vi "HEWH Extract Str Data.vi"(7 "Full Data (String)":string[][](array[string]), 8 "error in (no error)":errorcluster, 11 "UEF Calculated Values Input in":T1 {"Data Indexes"."15 sec after Draw Index" format="%#.2f"; "Data Indexes"."15 sec after Draw Timestamp" format="%#.2f"; "Data Indexes"."Test Start Timestamp" format="%.2f"; "Data Indexes"."Test End Timestamp" format="%.2f"; "Data Indexes"."T0 Timestamp" format="%.2f"; "Data Indexes"."Tsf Timestamp" format="%.2f"; "Data Indexes"."Tsu0 Timestamp" format="%.2f"; "Data Indexes"."Tmax1 Timestamp" format="%.2f"; "Data Indexes"."Draw Index Timestamp" format="%#.2f"; "Data Indexes"."Non-Draw Timestamp" format="%#.2f"; "Data Indexes"."Heating Timestamp" format="%#.2f"; "Data Indexes"."Start Energy (BTU-Gas)" format="%.6f"; "Data Indexes"."Start Watt Hours" format="%.6f"; "Static Data"."V - Volume of Wh (True)" format="%.5f"; "Static Data"."T-Ambinet Nominal (°F)" format="%.5f"; "Static Data"."T-Inlet Setpoint (°F)" format="%.5f"; "Static Data"."T-Wh Setpoint (°F)" format="%.5f"; "Sampled Data"."Qe (Wh)" format="%.5f"; "Sampled Data"."Tau stby2 (hr)" format="%.5f"; "Sampled Data"."Tastby2 (°F)" format="%.5f"; "Sampled Data"."Qf (BTU)" format="%.5f"; "Sampled Data"."Qe (BTU)" format="%.5f"; "Sampled Data"."Tmax1 (°F)" format="%.5f"; "Sampled Data"."T0 (°F)" format="%.5f"; "Sampled Data"."Qr (BTU)" format="%.5f"; "Sampled Data"."T 24(°F)" format="%.5f"; "Sampled Data"."T astby(°F)" format="%.5f"; "Sampled Data"."T tstby(°F)" format="%.5f"; "Sampled Data"."T su0(°F)" format="%.5f"; "Sampled Data"."T suf(°F)" format="%.5f"; "Sampled Data"."Tau stby_1 (hr)" format="%.5f"; "Sampled Data"."Qsuf (BTU)" format="%.5f"; "Sampled Data"."Qsu0 (BTU)" format="%.5f"; "Calculated Values"."Draw Bonus Volume (gal)" format="%.6f"; "Calculated Values"."Adjustment Factor" format="%.6f"; "Calculated Values"."T*avg_del(n-1)" format="%.6f"; "Calculated Values"."T*min(n-1)" format="%.6f"; "Calculated Values"."T*avg_del(n)" format="%.6f"; "Calculated Values"."Vn" format="%.6f"; "Calculated Values"."Qdm (BTU)" format="%.6f"; "Calculated Values"."QHWD (BTU)" format="%.6f"; "Calculated Values"."QHW (BTU)" format="%.6f"; "Calculated Values"."UEF" format="%.6f"; "Calculated Values"."QHW67 (BTU)" format="%.6f"; "Calculated Values"."Qda (BTU)" format="%.6f"; "Calculated Values"."Qd (BTU)" format="%.6f"; "Calculated Values"."Q (BTU)" format="%.6f"; "Calculated Values"."UA (BTU/(hr*F))" format="%.6f"; "Calculated Values"."Qhr (BTU/hr)" format="%.6f"; "Calculated Values"."Qstby (BTU)" format="%.6f"; "Calculated Values"."nu_r" format="%.6f"; "Calculated Values"."CpUEF (BTU/(lb*F))" format="%.6f"; "Calculated Values"."rho_nu (lb/gal)" format="%.6f"; "Calculated Values"."V1- Vol (Gal)" format="%.6f"; "Calculated Values"."M cluster mass removed (lb)" format="%.6f"; "Calculated Values"."Cp theoretical (BTU/(lbm °F))" format="%.6f"; "Calculated Values"."Tin1 - Mean Inlet 1st Cluster (°F)" format="%.6f"; "Calculated Values"."Tdel1-Mean Outlet 1st Cluster(°F)" format="%.6f"; "Calculated Values"."Cp 24 (BTU/(lb*F))" format="%.6f"; "Calculated Values"."Cp standby (BTU/(lb*F))" format="%.6f"; "Calculated Values"."Cp2 (BTU/(lb*F))" format="%.6f"; "Calculated Values"."Cp1 (BTU/(lb*F))" format="%.6f"; "Calculated Values"."rho 24 (lb/gal)" format="%.6f"; "Calculated Values"."rho standby (lb/gal)" format="%.6f"; "Calculated Values"."rho 2 (lb/gal)" format="%.6f"; "Calculated Values"."Density of cold water All (lbm/gal)" format="%#.3g"; "Calculated Values"."CpHW (BTU/(lbm °F))" format="%#.3g"; "Calculated Values"."Density of hot water All (lbm/gal)" format="%#.3g"; "Calculated Values"."Mass of water All (lbm)" format="%#.3f"}) -> (0 "error out":errorcluster, 1 "Full Data (String) Out":string[][](array[string]), 3 "UEF Calculated Values Input out":T1 {"Data Indexes"."15 sec after Draw Index" format="%#.2f"; "Data Indexes"."15 sec after Draw Timestamp" format="%#.2f"; "Data Indexes"."Test Start Timestamp" format="%.2f"; "Data Indexes"."Test End Timestamp" format="%.2f"; "Data Indexes"."T0 Timestamp" format="%.2f"; "Data Indexes"."Tsf Timestamp" format="%.2f"; "Data Indexes"."Tsu0 Timestamp" format="%.2f"; "Data Indexes"."Tmax1 Timestamp" format="%.2f"; "Data Indexes"."Draw Index Timestamp" format="%#.2f"; "Data Indexes"."Non-Draw Timestamp" format="%#.2f"; "Data Indexes"."Heating Timestamp" format="%#.2f"; "Data Indexes"."Start Energy (BTU-Gas)" format="%.6f"; "Data Indexes"."Start Watt Hours" format="%.6f"; "Static Data"."V - Volume of Wh (True)" format="%.5f"; "Static Data"."T-Ambinet Nominal (°F)" format="%.5f"; "Static Data"."T-Inlet Setpoint (°F)" format="%.5f"; "Static Data"."T-Wh Setpoint (°F)" format="%.5f"; "Sampled Data"."Qe (Wh)" format="%.5f"; "Sampled Data"."Tau stby2 (hr)" format="%.5f"; "Sampled Data"."Tastby2 (°F)" format="%.5f"; "Sampled Data"."Qf (BTU)" format="%.5f"; "Sampled Data"."Qe (BTU)" format="%.5f"; "Sampled Data"."Tmax1 (°F)" format="%.5f"; "Sampled Data"."T0 (°F)" format="%.5f"; "Sampled Data"."Qr (BTU)" format="%.5f"; "Sampled Data"."T 24(°F)" format="%.5f"; "Sampled Data"."T astby(°F)" format="%.5f"; "Sampled Data"."T tstby(°F)" format="%.5f"; "Sampled Data"."T su0(°F)" format="%.5f"; "Sampled Data"."T suf(°F)" format="%.5f"; "Sampled Data"."Tau stby_1 (hr)" format="%.5f"; "Sampled Data"."Qsuf (BTU)" format="%.5f"; "Sampled Data"."Qsu0 (BTU)" format="%.5f"; "Calculated Values"."Draw Bonus Volume (gal)" format="%.6f"; "Calculated Values"."Adjustment Factor" format="%.6f"; "Calculated Values"."T*avg_del(n-1)" format="%.6f"; "Calculated Values"."T*min(n-1)" format="%.6f"; "Calculated Values"."T*avg_del(n)" format="%.6f"; "Calculated Values"."Vn" format="%.6f"; "Calculated Values"."Qdm (BTU)" format="%.6f"; "Calculated Values"."QHWD (BTU)" format="%.6f"; "Calculated Values"."QHW (BTU)" format="%.6f"; "Calculated Values"."UEF" format="%.6f"; "Calculated Values"."QHW67 (BTU)" format="%.6f"; "Calculated Values"."Qda (BTU)" format="%.6f"; "Calculated Values"."Qd (BTU)" format="%.6f"; "Calculated Values"."Q (BTU)" format="%.6f"; "Calculated Values"."UA (BTU/(hr*F))" format="%.6f"; "Calculated Values"."Qhr (BTU/hr)" format="%.6f"; "Calculated Values"."Qstby (BTU)" format="%.6f"; "Calculated Values"."nu_r" format="%.6f"; "Calculated Values"."CpUEF (BTU/(lb*F))" format="%.6f"; "Calculated Values"."rho_nu (lb/gal)" format="%.6f"; "Calculated Values"."V1- Vol (Gal)" format="%.6f"; "Calculated Values"."M cluster mass removed (lb)" format="%.6f"; "Calculated Values"."Cp theoretical (BTU/(lbm °F))" format="%.6f"; "Calculated Values"."Tin1 - Mean Inlet 1st Cluster (°F)" format="%.6f"; "Calculated Values"."Tdel1-Mean Outlet 1st Cluster(°F)" format="%.6f"; "Calculated Values"."Cp 24 (BTU/(lb*F))" format="%.6f"; "Calculated Values"."Cp standby (BTU/(lb*F))" format="%.6f"; "Calculated Values"."Cp2 (BTU/(lb*F))" format="%.6f"; "Calculated Values"."Cp1 (BTU/(lb*F))" format="%.6f"; "Calculated Values"."rho 24 (lb/gal)" format="%.6f"; "Calculated Values"."rho standby (lb/gal)" format="%.6f"; "Calculated Values"."rho 2 (lb/gal)" format="%.6f"; "Calculated Values"."Density of cold water All (lbm/gal)" format="%#.3g"; "Calculated Values"."CpHW (BTU/(lbm °F))" format="%#.3g"; "Calculated Values"."Density of hot water All (lbm/gal)" format="%#.3g"; "Calculated Values"."Mass of water All (lbm)" format="%#.3f"})   [LabVIEW 2023]
uses:
  Type Definitions/UEF Constants.ctl
  Type Definitions/HEWH Draw Stats.ctl
  Type Definitions/HEWH FHR Draw Type.ctl
  Type Definitions/FHR Bins.ctl
  Type Definitions/HEWH Meter Type.ctl
panel:
  # "FHR"
  # "FHR"
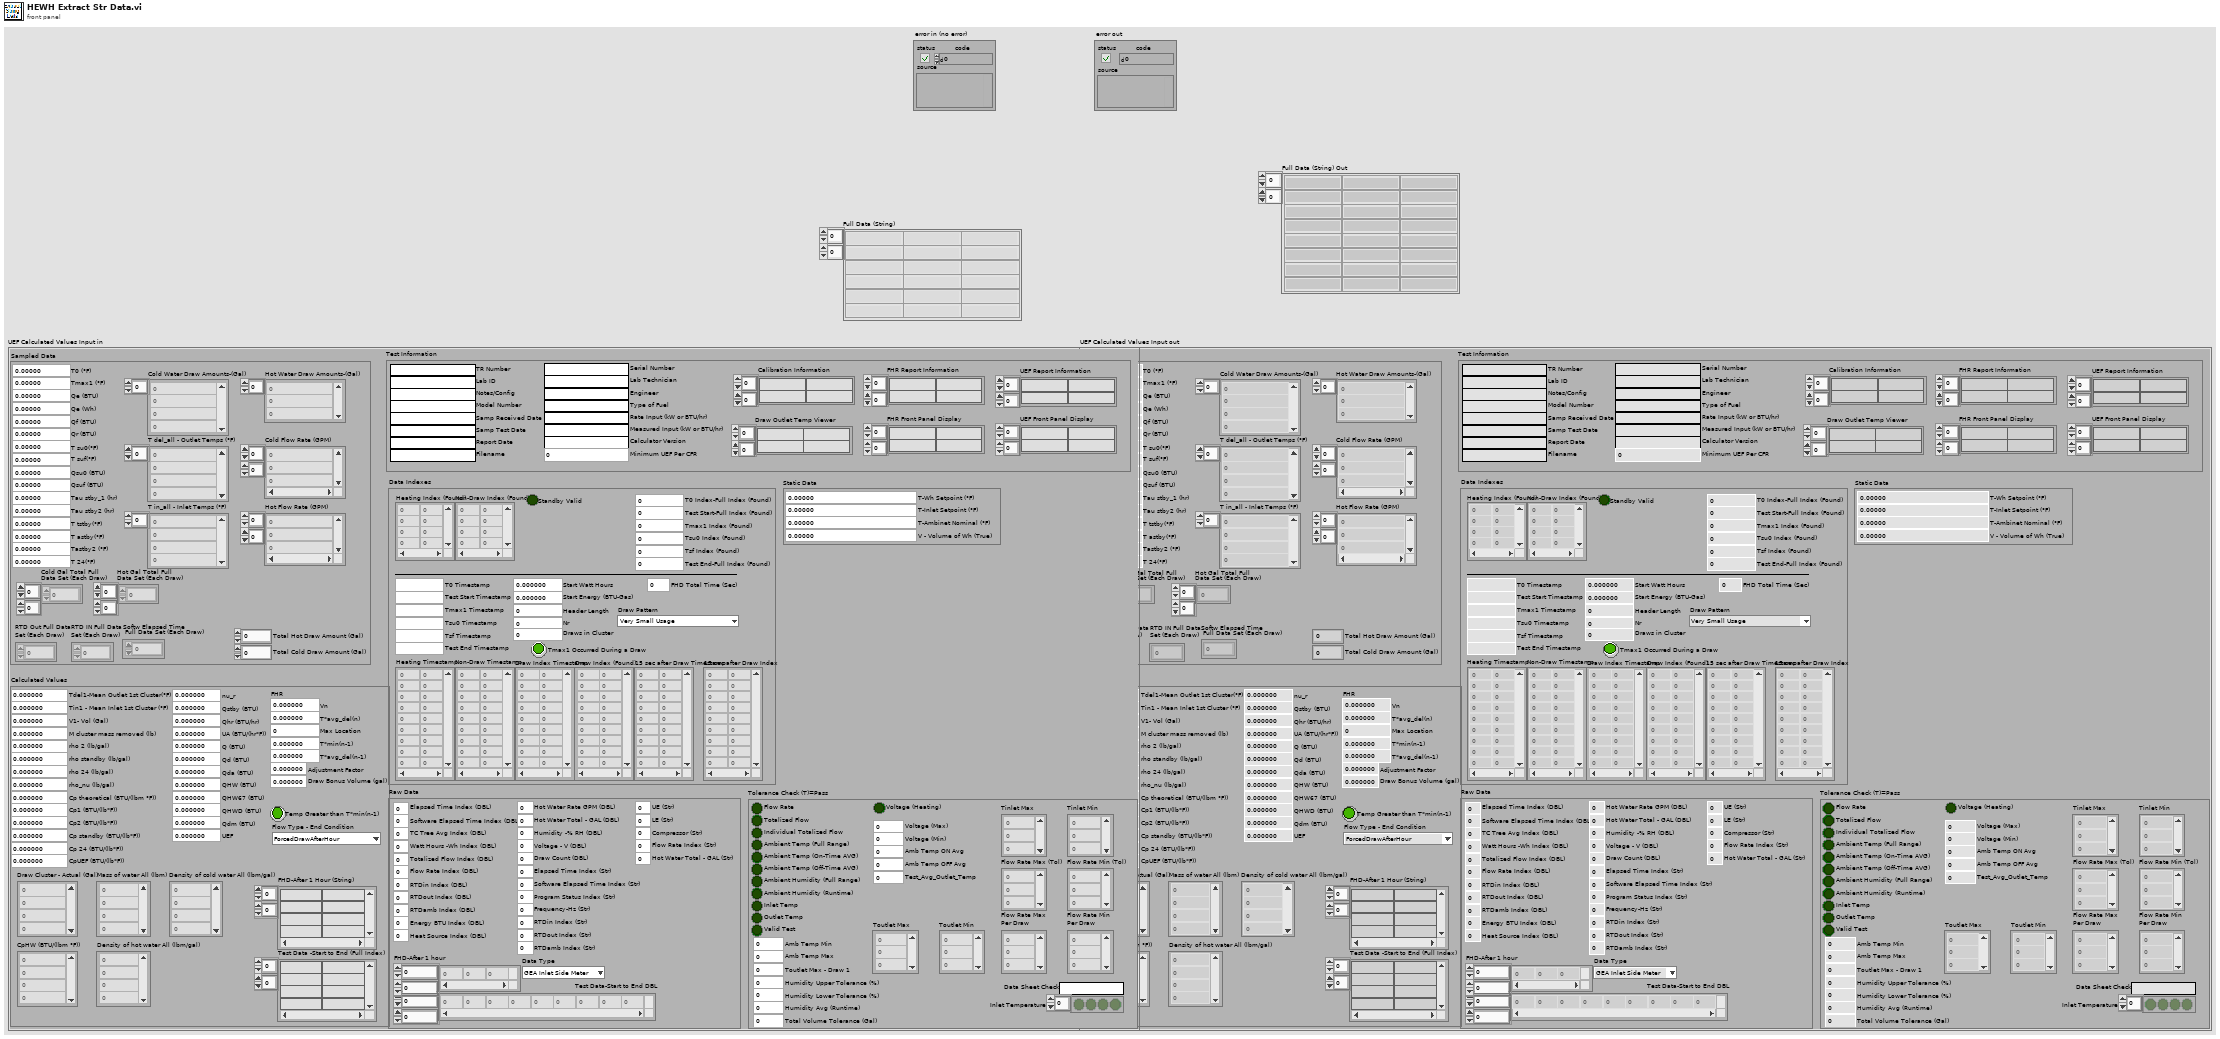
[diagram p1: front panel]
types:
  T1 = typedef "UEF Constants.ctl" = cluster{"Calculated Values":T2, "Sampled Data":cluster{"Cold Water Draw Amounts-(Gal)":dbl[], "T del_all - Outlet Temps (°F)":dbl[], "T in_all - Inlet Temps (°F)":dbl[], "Qsu0 (BTU)":dbl, "Qsuf (BTU)":dbl, "Tau stby_1 (hr)":dbl, "T suf(°F)":dbl, "T su0(°F)":dbl, "T tstby(°F)":dbl, "T astby(°F)":dbl, "T 24(°F)":dbl, "Qr (BTU)":dbl, "T0 (°F)":dbl, "Tmax1 (°F)":dbl, "Qe (BTU)":dbl, "Qf (BTU)":dbl, "Tastby2 (°F)":dbl, "RTD Out Full Data\nSet (Each Draw)":dbl[][], "RTD IN Full Data\nSet (Each Draw)":dbl[][], "Tau stby2 (hr)":dbl, "Hot Water Draw Amounts-(Gal)":dbl[], "Cold Flow Rate (GPM)":dbl[][], "Hot Flow Rate (GPM)":dbl[][], "Softw Elapsed Time\n Full Data Set (Each Draw)":dbl[][], "Cold Gal Total Full\nData Set (Each Draw)":dbl[][], "Total Hot Draw Amount (Gal) ":dbl, "Total Cold Draw Amount (Gal)":dbl, "Qe (Wh)":dbl, "Hot Gal Total Full\nData Set (Each Draw)":dbl[][]}, "Static Data":cluster{"T-Wh Setpoint (°F)":dbl, "T-Inlet Setpoint (°F)":dbl, "T-Ambinet Nominal (°F)":dbl, "V - Volume of Wh (True)":dbl}, "Data Indexes":cluster{"Test Start-Full Index (Found)":i32, "Header Length":i32, "Draw Index (Found)":i32[][], "Nr":i32, "Start Watt Hours":dbl, "Tsu0 Index (Found)":i32, "Tsf Index (Found)":i32, "Start Energy (BTU-Gas)":dbl, "Draws in Cluster":i32, "T0 Index-Full Index (Found)":i32, "Non-Draw Index (Found)":i32[][], "Tmax1 Index (Found)":i32, "Test End-Full Index (Found)":i32, "Heating Index (Found)":i32[][], "Heating Timestamp":dbl[][], "Non-Draw Timestamp":dbl[][], "Draw Index Timestamp":dbl[][], "Tmax1 Timestamp":dbl, "Tsu0 Timestamp":dbl, "Tsf Timestamp":dbl, "T0 Timestamp":dbl, "Test End Timestamp":dbl, "Test Start Timestamp":dbl, "15 sec after Draw Timestamp":dbl[][], "15 sec after Draw Index":dbl[][], "Tmax1 Occurred During a Draw":bool, "FHD Total Time (Sec)":dbl, "Draw Pattern":T4, "Standby Valid":bool}, "Raw Data":cluster{"Elapsed Time Index (DBL)":i32, "Software Elapsed Time Index (DBL)":i32, "TC Tree Avg Index (DBL)":i32, "Watt Hours -Wh Index (DBL)":i32, "Energy BTU Index (DBL)":i32, "Totalized Flow Index (DBL)":i32, "Flow Rate Index (DBL)":i32, "Program Status Index (Str)":i32, "RTDin Index (DBL)":i32, "RTDout Index (DBL)":i32, "RTDamb Index (DBL)":i32, "Test Data-Start to End DBL":dbl[][], "Data Type":T5, "Heat Source Index (DBL)":i32, "Hot Water Rate GPM (DBL)":i32, "Hot Water Total - GAL (DBL)":i32, "FHD-After 1 hour":dbl[][], "Humidity -% RH (DBL)":i32, "Voltage - V (DBL)":i32, "Draw Count (DBL)":i32, "Elapsed Time Index (Str)":i32, "Software Elapsed Time Index (Str)":i32, "Frequency-Hz (Str)":i32, "RTDin Index (Str)":i32, "RTDout Index (Str)":i32, "RTDamb Index (Str)":i32, "UE (Str)":i32, "LE (Str)":i32, "Compressor (Str)":i32, "Flow Rate Index (Str)":i32, "Hot Water Total - GAL (Str)":i32}, "Tolerance Check (T)=Pass":cluster{"Flow Rate":bool, "Totalized Flow":bool, "Ambient Temp (Full Range)":bool, "Ambient Humidity (Full Range)":bool, "Inlet Temp":bool, "Outlet Temp":bool, "Valid Test":bool, "Individual Totalized Flow":bool, "Data Sheet Check":string, "Inlet Temperature":bool[], "Tinlet Max":dbl[], "Tinlet Min":dbl[], "Flow Rate Max (Tol)":dbl[], "Flow Rate Min (Tol)":dbl[], "Amb Temp Max":dbl, "Amb Temp Min":dbl, "Toutlet Max - Draw 1":dbl, "Humidity Upper Tolerance (%)":dbl, "Total Volume Tolerance (Gal)":dbl, "Humidity Lower Tolerance (%)":dbl, "Flow Rate Max\nPer Draw":dbl[], "Flow Rate Min\nPer Draw":dbl[], "Ambient Humidity (Runtime)":bool, "Humidity Avg (Runtime)":dbl, "Ambient Temp (On-Time AVG)":bool, "Ambient Temp (Off-Time AVG)":bool, "Amb Temp OFF Avg":dbl, "Amb Temp ON Avg":dbl, "Voltage (Heating)":bool, "Voltage (Min)":dbl, "Voltage (Max)":dbl, "Toutlet Max":dbl[], "Toutlet Min":dbl[], "Test_Avg_Outlet_Temp":dbl}, "Test Information":cluster{"TR Number":string, "Lab ID":string, "Notes/Config":string, "Model Number":string, "Serial Number":string, "Lab Technician":string, "Engineer":string, "Type of Fuel":string, "Samp Received Date":string, "Samp Test Date":string, "Report Date":string, "Rate Input (kW or BTU/hr)":string, "Measured Input (kW or BTU/hr)":string, "Filename":string, "Calibration Information":string[][], "Calculator Version":string, "Minimum UEF Per CFR":dbl, "UEF Report Information":string[][], "FHR Report Information":string[][], "FHR Front Panel Display":string[][], "UEF Front Panel Display":string[][], "Draw Outlet Temp Viewer":string[][]}}
  T2 = typedef "HEWH Draw Stats.ctl" = cluster{"Draw Cluster - Actual (Gal)":dbl[], "Mass of water All (lbm)":dbl[], "Density of hot water All (lbm/gal)":dbl[], "CpHW (BTU/(lbm °F))":dbl[], "rho 2 (lb/gal)":dbl, "rho standby (lb/gal)":dbl, "rho 24 (lb/gal)":dbl, "Cp1 (BTU/(lb*F))":dbl, "Cp2 (BTU/(lb*F))":dbl, "Cp standby (BTU/(lb*F))":dbl, "Cp 24 (BTU/(lb*F))":dbl, "nu_r":dbl, "Qstby (BTU)":dbl, "Qhr (BTU/hr)":dbl, "UA (BTU/(hr*F))":dbl, "Q (BTU)":dbl, "Qd (BTU)":dbl, "Qda (BTU)":dbl, "QHW67 (BTU)":dbl, "UEF":dbl, "Tdel1-Mean Outlet 1st Cluster(°F)":dbl, "Tin1 - Mean Inlet 1st Cluster (°F)":dbl, "Cp theoretical (BTU/(lbm °F))":dbl, "M cluster mass removed (lb)":dbl, "V1- Vol (Gal)":dbl, "Test Data -Start to End (Full Index)":string[][], "rho_nu (lb/gal)":dbl, "Density of cold water All (lbm/gal)":dbl[], "CpUEF (BTU/(lb*F))":dbl, "QHW (BTU)":dbl, "QHWD (BTU)":dbl, "Qdm (BTU)":dbl, "FHD-After 1 Hour (String)":string[][], "Vn":dbl, "T*avg_del(n)":dbl, "Max Location":i32, "T*min(n-1)":dbl, "T*avg_del(n-1)":dbl, "Temp Greater than T*min(n-1)":bool, "Adjustment Factor":dbl, "Draw Bonus Volume (gal)":dbl, "Flow Type - End Condition":T3}
  T3 = typedef "HEWH FHR Draw Type.ctl" = enum16{"ForcedDrawAfterHour", "HeatingCutoffBeforeHour"}
  T4 = typedef "FHR Bins.ctl" = enum16{"Very Small Usage", "Low Usage", "Medium Usage", "High Usage", "Undefined"}
  T5 = typedef "HEWH Meter Type.ctl" = enum16{"GEA Inlet Side Meter", "GEA Outlet Side Meter", "CSA Inlet Side Meter"}
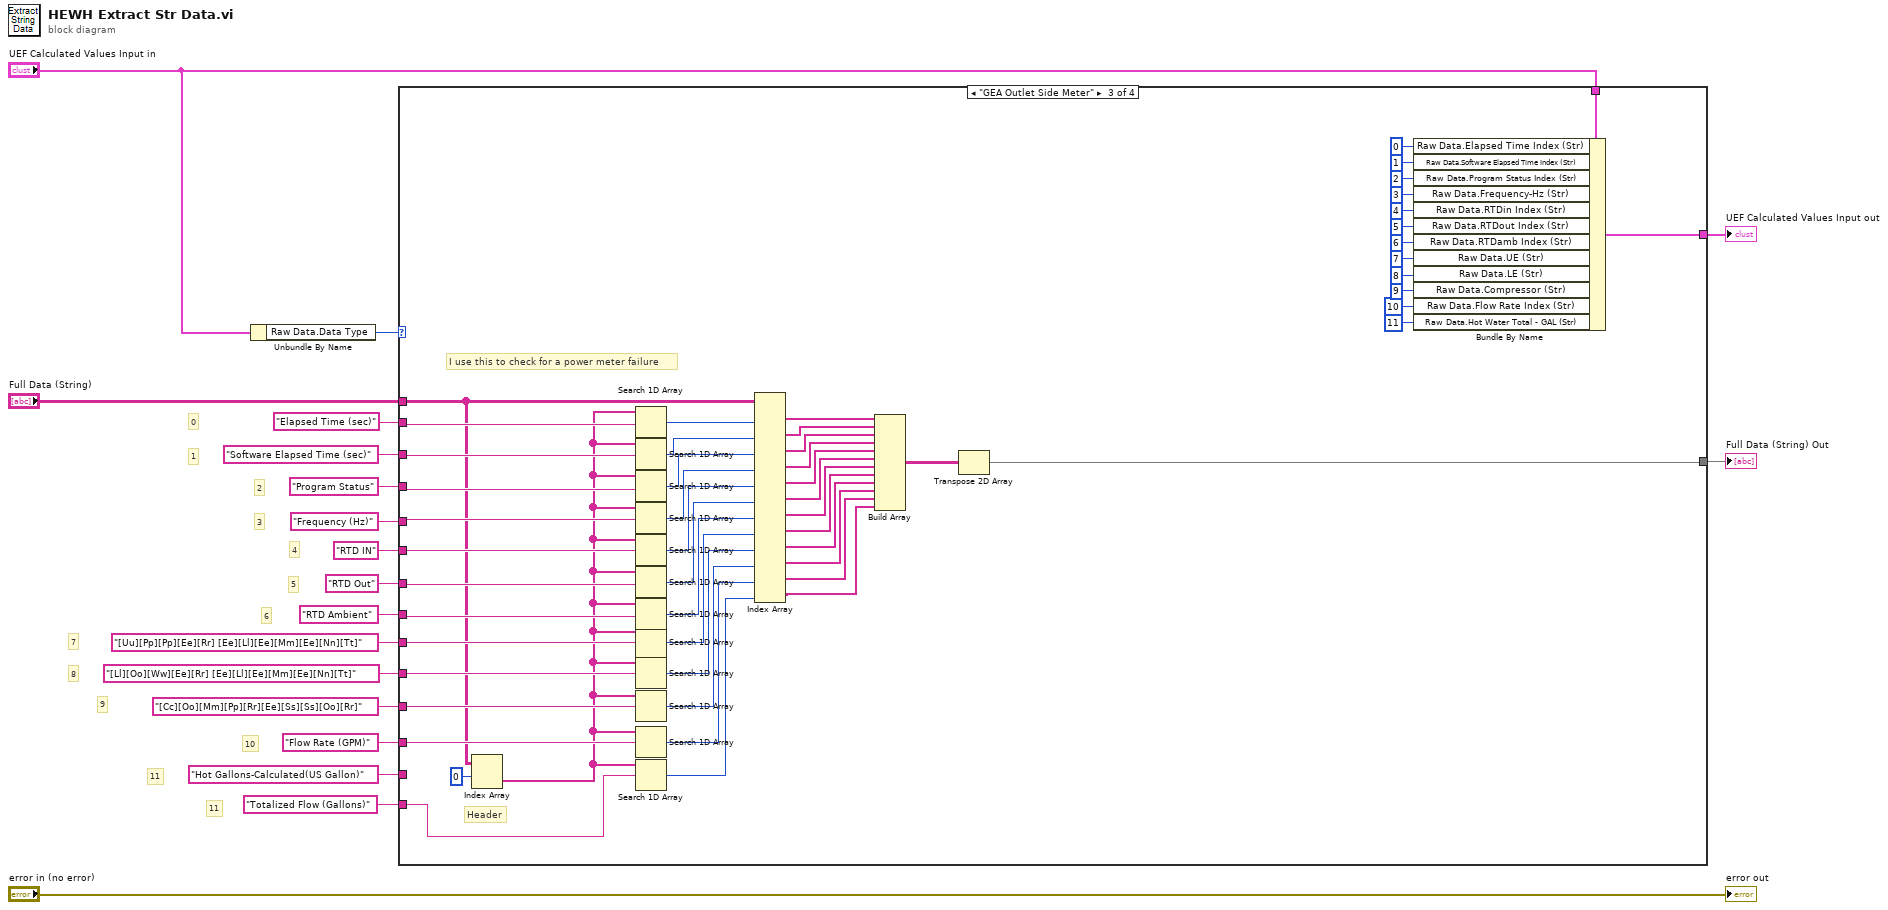
[diagram p0: block diagram]
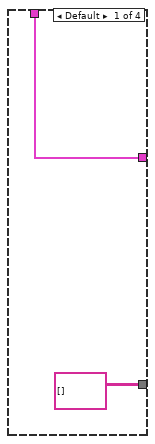
[diagram p2: hidden frame]
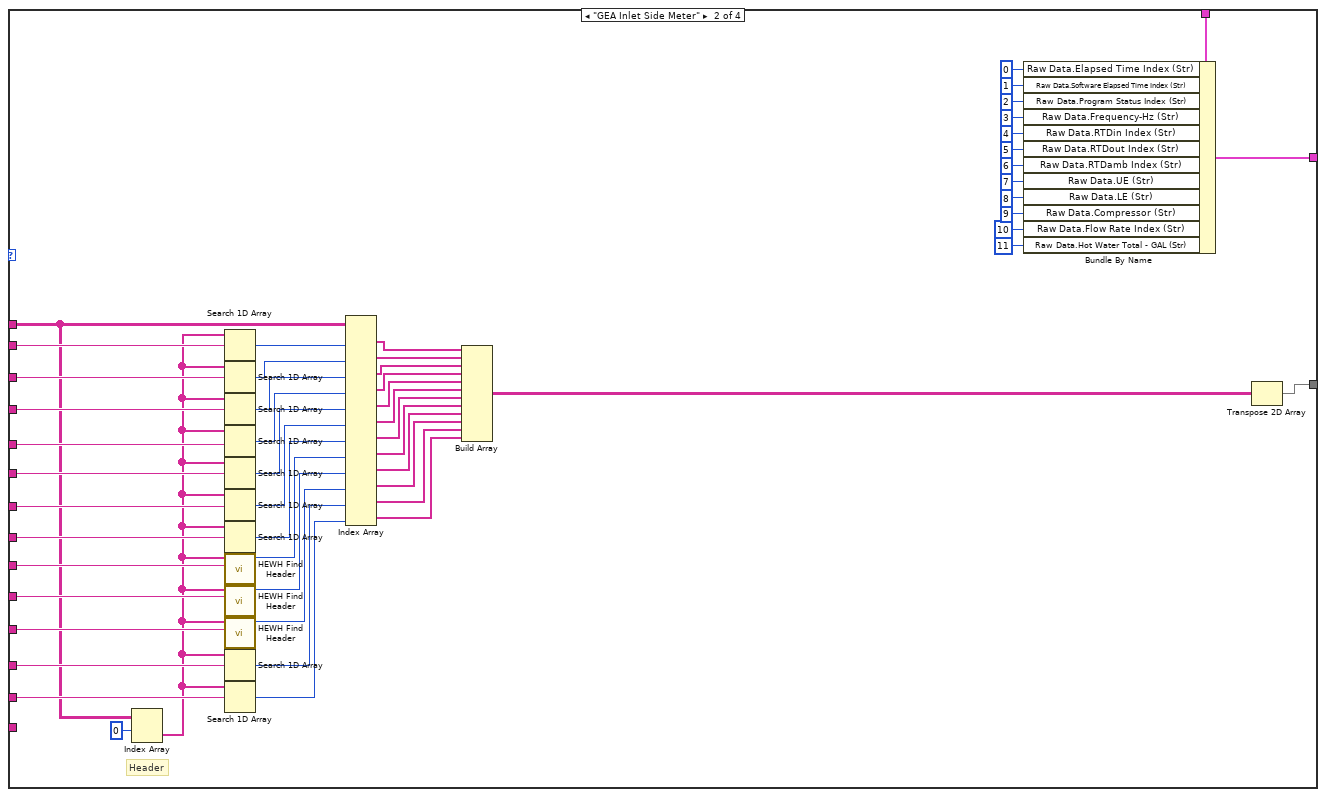
[diagram p3: hidden frame]
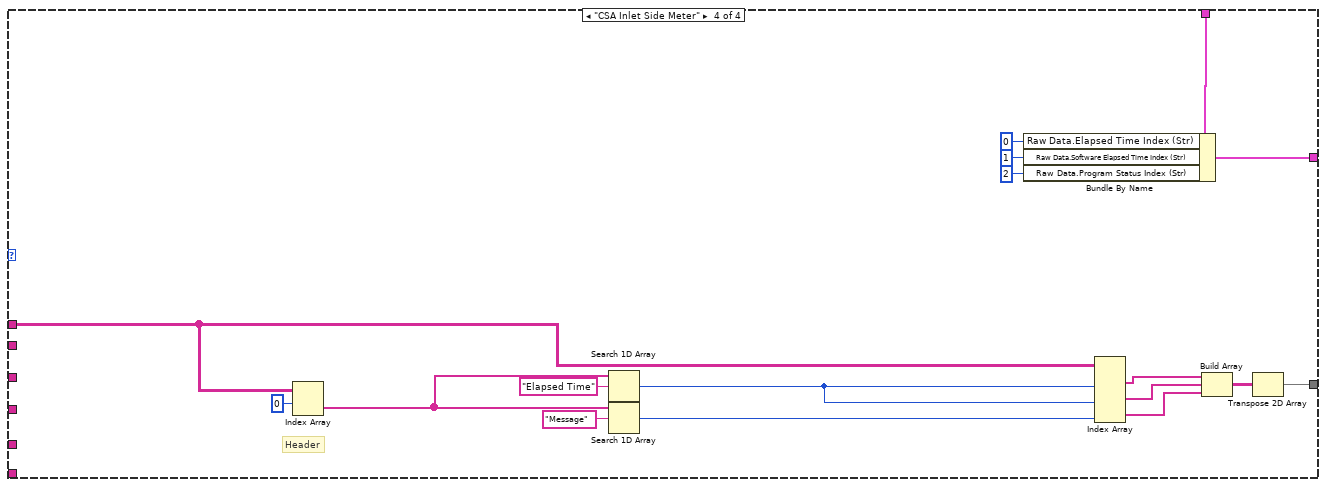
[diagram p4: hidden frame]
diagram:
  # "11"
  # "11"
  # "10"
  # "9"
  # "8"
  # "7"
  # "6"
  # "5"
  # "4"
  # "3"
  # "2"
  # "1"
  # "0"
  n1 = Unbundle By Name("UEF Calculated Values Input in") -> ("Raw Data.Data Type"=w3:T5)
  n2 = case shown="\"GEA Outlet Side Meter\"" w3 {
    tunnel: "Full Data (String)" -> [_ w32 w95 w132]
    tunnel: [string[][] [] w73 w126 w148] -> w18
    tunnel: "Elapsed Time (sec)" ("regular expression") -> [_ w50 w115 _]
    tunnel: "Software Elapsed Time (sec)" ("regular expression") -> [_ w49 w114 _]
    tunnel: "Program Status" ("regular expression") -> [_ w48 w113 _]
    tunnel: "Frequency (Hz)" ("regular expression") -> [_ w47 w112 _]
    tunnel: "RTD IN" ("regular expression") -> [_ w46 w111 _]
    tunnel: "RTD Out" ("regular expression") -> [_ w45 w110 _]
    tunnel: "RTD Ambient" ("regular expression") -> [_ w44 w109 _]
    tunnel: "[Uu][Pp][Pp][Ee][Rr] [Ee][Ll][Ee][Mm][Ee][Nn][Tt]" ("Expression") -> [_ w43 w108 _]
    tunnel: "[Ll][Oo][Ww][Ee][Rr] [Ee][Ll][Ee][Mm][Ee][Nn][Tt]" ("regular expression") -> [_ w42 w107 _]
    tunnel: "[Cc][Oo][Mm][Pp][Rr][Ee][Ss][Ss][Oo][Rr]" ("regular expression") -> [_ w41 w106 _]
    tunnel: "Flow Rate (GPM)" ("regular expression") -> [_ w40 w105 _]
    tunnel: "Hot Gallons-Calculated(US Gallon)" ("regular expression") -> [_ w39 _ _]
    tunnel: "UEF Calculated Values Input in" -> [w20 w35 w82 w136]
    tunnel: [w20 w34 w81 w135] -> w19
    tunnel: "Totalized Flow (Gallons)" ("regular expression") -> [_ _ w79 _]
    frame Default {
    }
    frame "GEA Inlet Side Meter" {
      # "Header"
      n3 = Index Array(array=w32, index (row)=0) -> (element=w31:string[])  [unwired: 1 in]
      n4 = Search 1D Array(1D array=w31, element=w50) -> (index of element=w59:i32)  [unwired: 1 in]
      n5 = Search 1D Array(1D array=w31, element=w49) -> (index of element=w58:i32)  [unwired: 1 in]
      n6 = Search 1D Array(1D array=w31, element=w48) -> (index of element=w72:i32)  [unwired: 1 in]
      n7 = Search 1D Array(1D array=w31, element=w47) -> (index of element=w70:i32)  [unwired: 1 in]
      n8 = Search 1D Array(1D array=w31, element=w46) -> (index of element=w60:i32)  [unwired: 1 in]
      n9 = Search 1D Array(1D array=w31, element=w45) -> (index of element=w56:i32)  [unwired: 1 in]
      n10 = Search 1D Array(1D array=w31, element=w44) -> (index of element=w55:i32)  [unwired: 1 in]
      n11 = call "HEWH Find Header.vi"("Expression"=w43, "Header"=w31) -> ("Index"=w54:i32)  [unwired: 9 in]
      n12 = call "HEWH Find Header.vi"("Expression"=w42, "Header"=w31) -> ("Index"=w53:i32)  [unwired: 9 in]
      n13 = call "HEWH Find Header.vi"("Expression"=w41, "Header"=w31) -> ("Index"=w52:i32)  [unwired: 9 in]
      n14 = Search 1D Array(1D array=w31, element=w40) -> (index of element=w57:i32)  [unwired: 1 in]
      n15 = Search 1D Array(1D array=w31, element=w39) -> (index of element=w51:i32)  [unwired: 1 in]
      n16 = Index Array(array=w32, index (col) #1=w59, index (col) #2=w58, index (col) #3=w72, index (col) #4=w70, index (col) #5=w60, index (col) #6=w56, index (col) #7=w55, index (col) #8=w54, index (col) #9=w53, index (col) #10=w52, index (col) #11=w57, index (col) #12=w51) -> (element #1=w74:string[], element #2=w75:string[], element #3=w71:string[], element #4=w69:string[], element #5=w68:string[], element #6=w67:string[], element #7=w66:string[], element #8=w65:string[], element #9=w64:string[], element #10=w63:string[], element #11=w62:string[], element #12=w61:string[])  [unwired: 12 in]
      n17 = Build Array(w74, w75, w71, w69, w68, w67, w66, w65, w64, w63, w62, w61) -> (w76:string[][])
      n18 = Bundle By Name(cluster=w35, "Raw Data.Elapsed Time Index (Str)"=0 ("Raw Data.Elapsed Time Index"), "Raw Data.Software Elapsed Time Index (Str)"=1 ("Raw Data.Elapsed Time Index"), "Raw Data.Program Status Index (Str)"=2 ("Raw Data.Elapsed Time Index"), "Raw Data.Frequency-Hz (Str)"=3 ("Raw Data.Elapsed Time Index"), "Raw Data.RTDin Index (Str)"=4 ("Raw Data.Elapsed Time Index"), "Raw Data.RTDout Index (Str)"=5 ("Raw Data.Elapsed Time Index"), "Raw Data.RTDamb Index (Str)"=6 ("Raw Data.Elapsed Time Index"), "Raw Data.UE (Str)"=7 ("Raw Data.Elapsed Time Index"), "Raw Data.LE (Str)"=8 ("Raw Data.Elapsed Time Index"), "Raw Data.Compressor (Str)"=9 ("Raw Data.Elapsed Time Index"), "Raw Data.Flow Rate Index (Str)"=10 ("Raw Data.Elapsed Time Index"), "Raw Data.Hot Water Total - GAL (Str)"=11 ("Raw Data.Elapsed Time Index")) -> (w34:T1)
      n19 = Transpose 2D Array(2D array=w76) -> (transposed array=w73:string[][])
    }
    frame "GEA Outlet Side Meter" {
      # "I use this to check for a power meter failure"
      # "Header"
      n20 = Index Array(array=w95, index (row)=0) -> (element=w80:string[])  [unwired: 1 in]
      n21 = Search 1D Array(1D array=w80, element=w115) -> (index of element=w120:i32)  [unwired: 1 in]
      n22 = Search 1D Array(1D array=w80, element=w114) -> (index of element=w119:i32)  [unwired: 1 in]
      n23 = Search 1D Array(1D array=w80, element=w113) -> (index of element=w128:i32)  [unwired: 1 in]
      n24 = Search 1D Array(1D array=w80, element=w112) -> (index of element=w121:i32)  [unwired: 1 in]
      n25 = Search 1D Array(1D array=w80, element=w111) -> (index of element=w118:i32)  [unwired: 1 in]
      n26 = Search 1D Array(1D array=w80, element=w110) -> (index of element=w117:i32)  [unwired: 1 in]
      n27 = Search 1D Array(1D array=w80, element=w109) -> (index of element=w116:i32)  [unwired: 1 in]
      n28 = Search 1D Array(1D array=w80, element=w108) -> (index of element=w104:i32)  [unwired: 1 in]
      n29 = Search 1D Array(1D array=w80, element=w107) -> (index of element=w103:i32)  [unwired: 1 in]
      n30 = Search 1D Array(1D array=w80, element=w106) -> (index of element=w102:i32)  [unwired: 1 in]
      n31 = Search 1D Array(1D array=w80, element=w105) -> (index of element=w101:i32)  [unwired: 1 in]
      n32 = Search 1D Array(1D array=w80, element=w79) -> (index of element=w78:i32)  [unwired: 1 in]
      n33 = Index Array(array=w95, index (col) #1=w120, index (col) #2=w119, index (col) #3=w128, index (col) #4=w121, index (col) #5=w118, index (col) #6=w117, index (col) #7=w116, index (col) #8=w104, index (col) #9=w103, index (col) #10=w102, index (col) #11=w101, index (col) #12=w78) -> (element #1=w129:string[], element #2=w130:string[], element #3=w127:string[], element #4=w125:string[], element #5=w124:string[], element #6=w123:string[], element #7=w122:string[], element #8=w100:string[], element #9=w99:string[], element #10=w98:string[], element #11=w97:string[], element #12=w77:string[])  [unwired: 12 in]
      n34 = Build Array(w129, w130, w127, w125, w124, w123, w122, w100, w99, w98, w97, w77) -> (w131:string[][])
      n35 = Transpose 2D Array(2D array=w131) -> (transposed array=w126:string[][])
      n36 = Bundle By Name(cluster=w82, "Raw Data.Elapsed Time Index (Str)"=0 ("Raw Data.Elapsed Time Index"), "Raw Data.Software Elapsed Time Index (Str)"=1 ("Raw Data.Elapsed Time Index"), "Raw Data.Program Status Index (Str)"=2 ("Raw Data.Elapsed Time Index"), "Raw Data.Frequency-Hz (Str)"=3 ("Raw Data.Elapsed Time Index"), "Raw Data.RTDin Index (Str)"=4 ("Raw Data.Elapsed Time Index"), "Raw Data.RTDout Index (Str)"=5 ("Raw Data.Elapsed Time Index"), "Raw Data.RTDamb Index (Str)"=6 ("Raw Data.Elapsed Time Index"), "Raw Data.UE (Str)"=7 ("Raw Data.Elapsed Time Index"), "Raw Data.LE (Str)"=8 ("Raw Data.Elapsed Time Index"), "Raw Data.Compressor (Str)"=9 ("Raw Data.Elapsed Time Index"), "Raw Data.Flow Rate Index (Str)"=10 ("Raw Data.Elapsed Time Index"), "Raw Data.Hot Water Total - GAL (Str)"=11 ("Raw Data.Elapsed Time Index")) -> (w81:T1)
    }
    frame "CSA Inlet Side Meter" {
      # "Header"
      n37 = Index Array(array=w132, index (row)=0) -> (element=w133:string[])  [unwired: 1 in]
      n38 = Search 1D Array(1D array=w133, element="Elapsed Time" ("regular expression")) -> (index of element=w140:i32)  [unwired: 1 in]
      n39 = Search 1D Array(1D array=w133, element="Message" ("regular expression")) -> (index of element=w143:i32)  [unwired: 1 in]
      n40 = Bundle By Name(cluster=w136, "Raw Data.Elapsed Time Index (Str)"=0 ("Raw Data.Elapsed Time Index"), "Raw Data.Software Elapsed Time Index (Str)"=1 ("Raw Data.Elapsed Time Index"), "Raw Data.Program Status Index (Str)"=2 ("Raw Data.Elapsed Time Index")) -> (w135:T1)
      n41 = Index Array(array=w132, index (col) #1=w140, index (col) #2=w140, index (col) #3=w143) -> (element #1=w145:string[], element #2=w144:string[], element #3=w142:string[])  [unwired: 3 in]
      n42 = Build Array(w145, w144, w142) -> (w146:string[][])
      n43 = Transpose 2D Array(2D array=w146) -> (transposed array=w148:string[][])
    }
  }
  "UEF Calculated Values Input out" <- w19
  "Full Data (String) Out" <- w18
  "error out" <- "error in (no error)"
